vi "dfd_DFXP Max and Min.vi"(8 "Word Length":i16) -> (1 "Minimum":i64 format="%.0x", 2 "Maximum":i64 format="%.0x")   [LabVIEW 2017, in "NI_DigFilter_FXP.lvlib"]
uses:
  <vilib>/addons/Digital Filter Design/NI_DigFilter_FXP.lvlib
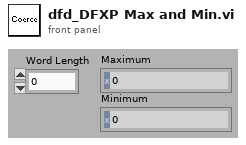
[diagram p1: front panel]
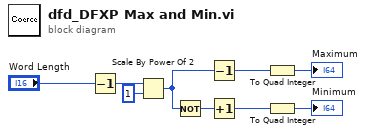
[diagram p0: block diagram]
diagram:
  n1 = Decrement(x="Word Length") -> (x-1=w3:i16)
  n2 = Scale By Power Of 2(n=w3, x=u64 1) -> (x*2^n=w1:u64)
  n3 = Not(x=w1) -> (.not. x?=w2:u64)
  n4 = Decrement(x=w1) -> (x-1=w8:u64)
  n5 = Increment(x=w2) -> (x+1=w9:u64)
  n6 = To Quad Integer(1:w8) -> (0:→"Maximum":i64)
  n7 = To Quad Integer(1:w9) -> (0:→"Minimum":i64)
